vi "Calc Eval.vi"(8 "error in (no error)":errorcluster, 10 "Inputs":dbl[](array[numeric]), 11 "Median Calc in":refnum<class "Median Calc.lvclass">) -> (0 "error out":errorcluster, 1 "Additional Updates":T1[](array[typedef]), 2 "Result":dbl, 3 "Median Calc out":refnum<class "Median Calc.lvclass">)   [LabVIEW 2020, in "VolatusCalcs.lvlib" / "Median Calc.lvclass"]
uses:
  Median Calc.lvclass
  Median Calc.lvclass/Median Calc.ctl
  <vilib>/Analysis/NI_AALBase.lvlib
  Calculation/Additional Update.ctl
  Calculation/Calculation.lvclass
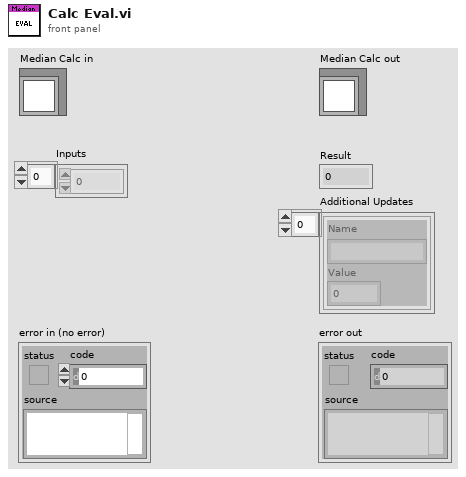
[diagram p1: front panel]
types:
  T1 = typedef "VolatusCalcs.lvlib/Calculation.lvclass/Additional Update.ctl" = cluster{"Name":string, "Value":dbl}
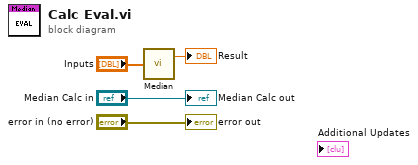
[diagram p0: block diagram]
diagram:
  n1 = call <vilib>:"Median.vi"("X"="Inputs") -> ("median"=→"Result":dbl)  [unwired: 1 out]
  "error out" <- "error in (no error)"
  "Median Calc out" <- "Median Calc in"
